vi "Write Last Known State.vi"(8 "error in (no error)":errorcluster, 11 "FP-TC-Shared in":refnum<class "FP-TC-Shared.lvclass">) -> (0 "error out":errorcluster, 3 "FP-TC-Shared out":refnum<class "FP-TC-Shared.lvclass">)   [LabVIEW 2019, in "FP-TC-Shared.lvclass"]
uses:
  FP-TC-Shared.lvclass
  <userlib>/LevyLab/Configuration/Configuration.lvclass
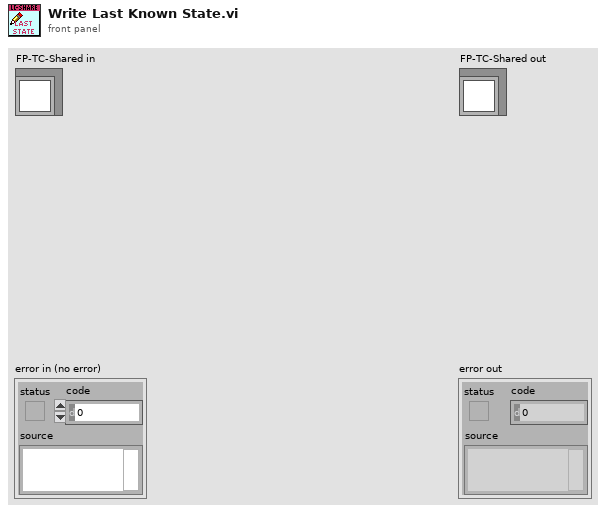
[diagram p1: front panel]
types:
  T1 = typedef "FP-TC-Shared.lvclass/LC Type--Enum.ctl" = enum16{"CF.TC", "CF.TC.Z", "CF.FP", "MNK.TC", "MNK.TC.Z", "MNK.FP"}
  T2 = cluster{"Application":enum16{"TC", "FP"}, "LC Type":T1}
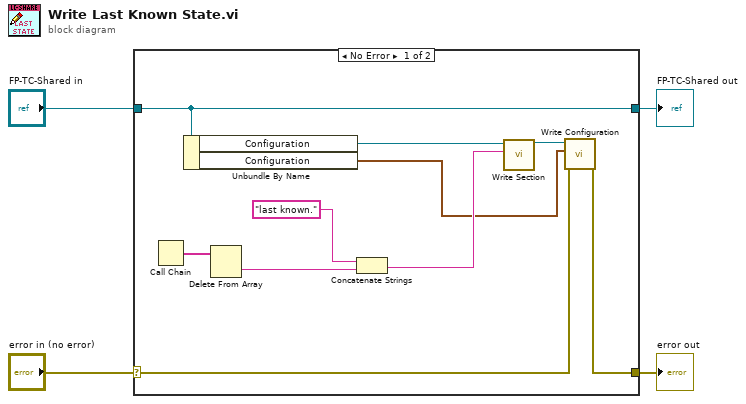
[diagram p0: block diagram]
diagram:
  n1 = case shown="No Error" "error in (no error)" {
    selector: "error in (no error)" -> [w7 w16]
    tunnel: [w6 w16] -> w3
    tunnel: [w11 w15] -> w1
    tunnel: "FP-TC-Shared in" -> [w11 w15]
    frame No Error {
      n2 = Call Chain() -> (call chain=w14:string[])
      n3 = Unbundle By Name(w11) -> ("Configuration"=w10:refnum<class "Configuration.lvclass">, "Configuration"=w5:T2)
      n4 = Delete From Array(array=w14) -> (deleted portion=w12:string)  [unwired: 2 in, 1 out]
      n5 = Concatenate Strings("last known.", w12) -> (w9:string)
      n6 = call <userlib>:"Write Section.vi"("Section"=w9, "Configuration in"=w10) -> ("Configuration out"=w8:refnum<class "Configuration.lvclass">)  [unwired: 8 in, 1 out]
      n7 = call <userlib>:"Write Configuration.vi"("error in (no error)"=w7, "Variant"=w5, "Configuration in"=w8) -> ("error out"=w6:errorcluster)  [unwired: 7 in, 1 out]
    }
    frame Error {
    }
  }
  "error out" <- w3
  "FP-TC-Shared out" <- w1
